vi "Cal Inst - Take Electrical Measurements.vi"(8 "error in (no error)":errorcluster, 10 "Temperature in":dbl, 11 "VISA Refnum in":refnum<visa-resource-name>) -> (0 "error out":errorcluster, 2 "Electrical Data":T1, 3 "VISA Refnum out":refnum<visa-resource-name>)   [LabVIEW 2013]
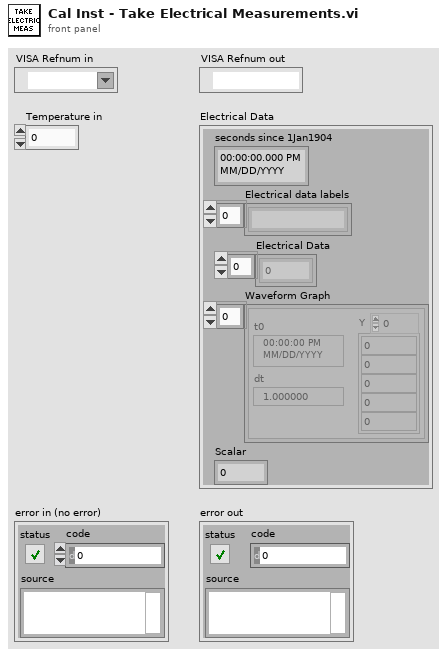
[diagram p1: front panel]
types:
  T1 = cluster{"seconds since 1Jan1904":timestamp, "Electrical data labels":string[], "Electrical Data":dbl[], "Waveform Graph":waveform(sgl)[], "Scalar":dbl}
  T2 = cluster{"seconds since 1Jan1904":timestamp, "Electrical data labels":string[], "Electrical Data":dbl[], "Waveform Graph":waveform(sgl)[], "Temperature in":dbl}
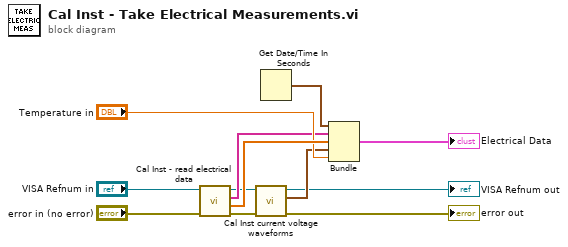
[diagram p0: block diagram]
diagram:
  n1 = call "Cal Inst - read electrical data.vi"("error in (no error)"="error in (no error)", "VISA Refnum in"="VISA Refnum in") -> ("error out"=w4:errorcluster, "Electrical Data"=w11:dbl[], "Electrical data labels"=w5:string[], "VISA Refnum out"=w2:refnum<visa-resource-name>)  [unwired: 6 in]
  n2 = call "Cal Inst current voltage waveforms.vi"("error in (no error)"=w4, "VISA resource name"=w2) -> ("error out"=→"error out":errorcluster, "Waveform Graph"=w6:waveform(sgl)[], "VISA resource name out"=→"VISA Refnum out":refnum<visa-resource-name>)  [unwired: 7 in]
  n3 = Get Date/Time In Seconds() -> (seconds since 1Jan1904=w12:timestamp)
  n4 = Bundle("seconds since 1Jan1904"=w12, "Electrical data labels"=w5, "Electrical Data"=w11, "Waveform Graph"=w6, "Temperature in"="Temperature in") -> (→"Electrical Data":T2)  [unwired: 1 in]
